vi "New Node.vi"(8 "error in (no error)":errorcluster, 10 "UID":string, 11 "Base Tree in":refnum<class "Base Tree.lvclass">) -> (0 "error out":errorcluster, 2 "Generic Node out":refnum<class "Generic Node.lvclass">, 3 "Base Tree out":refnum<class "Base Tree.lvclass">)   [LabVIEW 2017, in "Browser Core.lvlib" / "Base Tree.lvclass"]
doc: "Create new Node Class from UID Input"
uses:
  Base Tree.lvclass
  Node Classes/Generic Node/Generic Node.lvclass
  Node Classes/Generic Node/Generic Node.lvclass/Generic Node.ctl
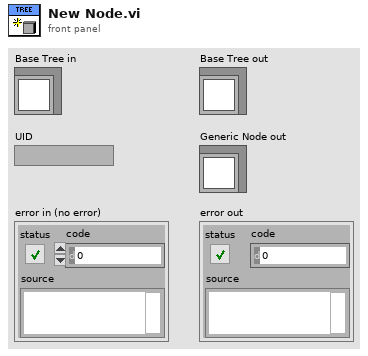
[diagram p1: front panel]
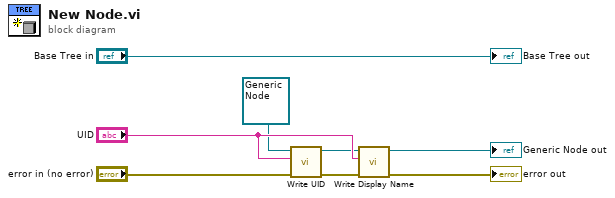
[diagram p0: block diagram]
diagram:
  n1 = call "Write UID.vi"("error in (no error)"="error in (no error)", "UID"="UID", "Generic Node in"=refnum<class "Generic Node.lvclass"> refnum ("New Node")) -> ("error out"=w1:errorcluster, "Generic Node out"=w2:refnum<class "Generic Node.lvclass">)  [unwired: 7 in]
  n2 = call "Write Display Name.vi"("error in (no error)"=w1, "Display Name"="UID", "Generic Node in"=w2) -> ("error out"=→"error out":errorcluster, "Generic Node out"=→"Generic Node out":refnum<class "Generic Node.lvclass">)  [unwired: 7 in]
  "Base Tree out" <- "Base Tree in"
